vi "AutoConfigureAdditionalMotionPlanes.vi"(0 "Motion ROIs":T2(array[cluster]), 1 "In Points":i32[][](array[numeric]), 3 "Grid Points":i32=10, 4 "Motion Rate (Hz)":dbl=10.0, 5 "error in (no error)":errorcluster, 6 "Number of Motion Points":i32, 7 "Scan Settings":T1, 10 "Plane Params":cluster{"Z Offset Per Box":i32, "Box Size":dbl}={"Z Offset Per Box"=6, "Box Size"=12.0}, 11 "Scan Settings (um)":T1={"XStart"=-100, "XEnd"=100, "XNum"=250, "YStart"=-100, "YEnd"=100, "YNum"=250, "ZStart"=-50, "ZEnd"=50, "ZNum"=30}) -> (12 "X-Y Motion Points":i32[][](array[numeric]), 13 "Y-Z Motion Points":i32[][](array[numeric]), 14 "Out Points":i32[][](array[numeric]), 15 "Total Motion Points":i32, 16 "Number of Motion Volumes":i32, 17 "Motion Increment":i32, 18 "Sampling Interval":dbl, 19 "error out":errorcluster)   [LabVIEW 2014]
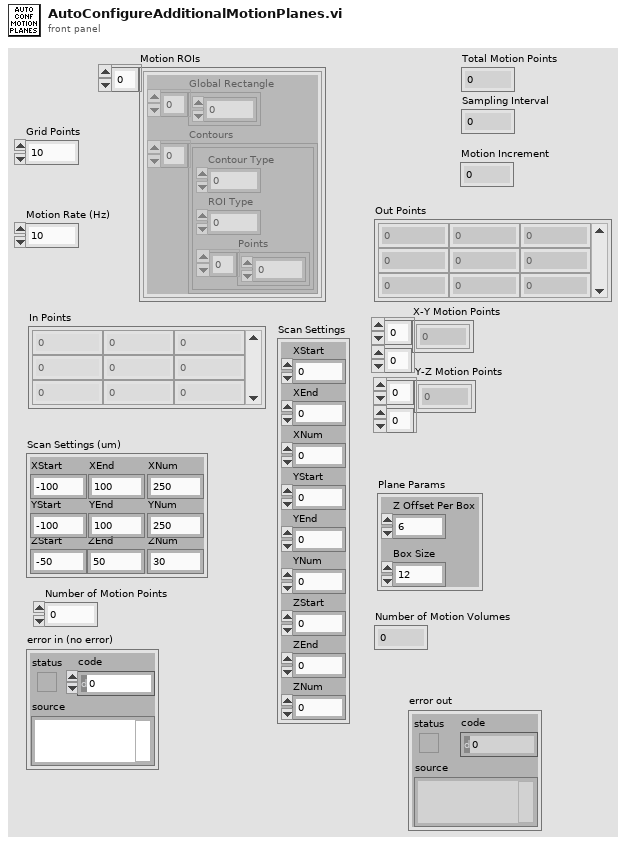
[diagram p1: front panel]
types:
  T1 = cluster{"XStart":i32, "XEnd":i32, "XNum":i32, "YStart":i32, "YEnd":i32, "YNum":i32, "ZStart":i32, "ZEnd":i32, "ZNum":i32}
  T2 = cluster{"Global Rectangle":i32[], "Contours":cluster{"Contour Type":u32, "ROI Type":u32, "Points":i32[]}[]}[]
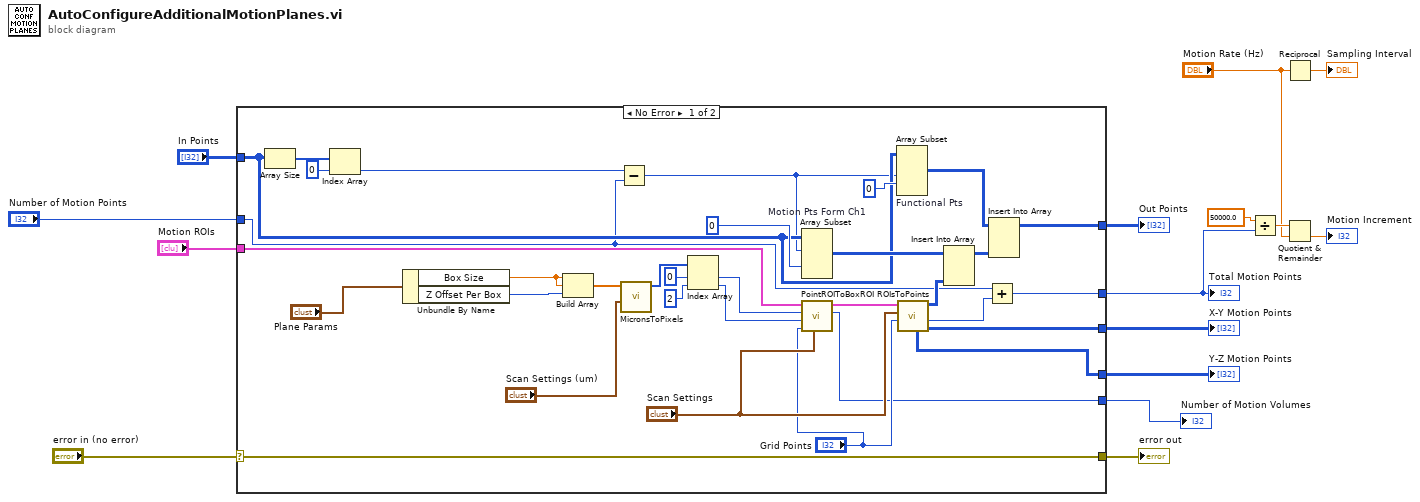
[diagram p0: block diagram]
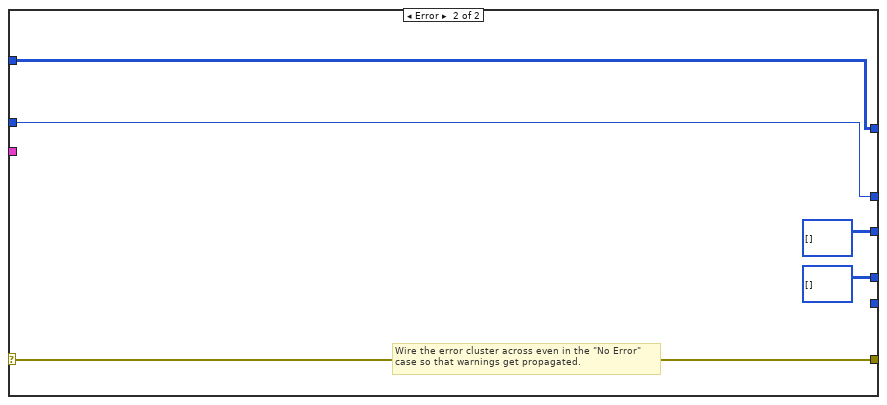
[diagram p2: hidden frame]
diagram:
  n1 = case shown="No Error" "error in (no error)" {
    selector: "error in (no error)" -> [w48 w53]
    tunnel: [w48 w53] -> w14
    tunnel: "Motion ROIs" -> [w47 _]
    tunnel: [w33 w52] -> w12
    tunnel: "In Points" -> [w32 w52]
    tunnel: [w30 w51] -> w8
    tunnel: "Number of Motion Points" -> [w29 w51]
    tunnel: [w27 i32[][] [] ("Y-Z Motion Points")] -> w3
    tunnel: [w26 i32[][] [] ("X-Y Motion Points")] -> w2
    tunnel: [w16 _] -> w1
    frame No Error {
      n2 = Array Size(array=w32) -> (size(s)=w42:i32[])
      n3 = Index Array(array=w42, index=0) -> (element=w40:i32)
      n4 = Unbundle By Name("Plane Params") -> ("Box Size"=w21:dbl, "Z Offset Per Box"=w23:i32)
      n5 = Build Array(w21, w21, w23) -> (w24:dbl[])
      n6 = Subtract(x=w40, y=w29) -> (x-y=w28:i32)
      n7 = call "MicronsToPixels.vi"("Scan Settings (um)"="Scan Settings (um)", "Microns (X,Y,Z)"=w24) -> ("Pixels (X,Y,Z)"=w46:i32[])  [unwired: 9 in]
      n8 = Index Array(array=w46, index #1=0 ("index"), index #2=2 ("index")) -> (element #1=w19:i32, element #2=w20:i32)
      n9 = Array Subset "Motion Pts Form Ch1"(array=w32, index (row)=w28, index (col)=0 ("index")) -> (w37:i32[][])  [unwired: 2 in]
      n10 = call "PointROIToBoxROI.vi"("Scan Settings"="Scan Settings", "Number of Boxes"="Grid Points", "Box Offset Z (pixels)"=w20, "Box Size (pixels)"=w19, "PT ROIs"=w47) -> ("Number of Motion Volumes"=w16:i32, "BOX ROIs"=w18:T2)  [unwired: 5 in]
      n11 = Array Subset "Functional Pts"(array=w32, length (row)=w28, index (col)=0 ("index")) -> (w35:i32[][])  [unwired: 2 in]
      n12 = call "ROIsToPoints.vi"("GridPoints"="Grid Points", "Scan Settings"="Scan Settings", "ROI"=w18) -> ("X-Y Motion Points"=w26:i32[][], "Number of motion points"=w31:i32, "Points"=w36:i32[][], "Y-Z Motion Points"=w27:i32[][])  [unwired: 4 in, 1 out]
      n13 = Insert Into Array(array=w37, new element=w36) -> (w34:i32[][])  [unwired: 2 in]
      n14 = Add(x=w29, y=w31) -> (x+y=w30:i32)
      n15 = Insert Into Array(array=w35, new element=w34) -> (w33:i32[][])  [unwired: 2 in]
    }
    frame Error {
      # "Wire the error cluster across even in the \"No Error\"\ncase so that warnings get propagated."
    }
  }
  "error out" <- w14
  "Out Points" <- w12
  "Total Motion Points" <- w8
  "X-Y Motion Points" <- w2
  "Y-Z Motion Points" <- w3
  "Number of Motion Volumes" <- w1
  n16 = Divide(x=50000.0, y=w8) -> (x/y=w7:dbl)
  n17 = Reciprocal(x="Motion Rate (Hz)") -> (1/x=→"Sampling Interval":dbl)
  n18 = Quotient & Remainder(x=w7, y="Motion Rate (Hz)") -> (floor(x/y)=→"Motion Increment":dbl)  [unwired: 1 out]
